vi "HP81110A Transfer String Into Memory.vi"(8 "error in (no error)":errorcluster, 9 "String":string, 10 "Channel (1:Channel 1)":T1(ring)=enum."Channel 1", 11 "VISA session":refnum<visa-resource-name>) -> (0 "error out":errorcluster, 2 "length":i32, 3 "dup VISA session":refnum<visa-resource-name>)   [LabVIEW 2023]
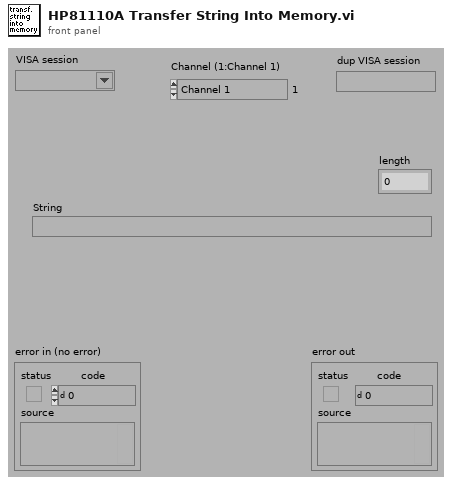
[diagram p1: front panel]
types:
  T1 = enum16{"Channel All ", "Channel 1", "Channel 2", "Channel 3", "Channels Combined"}
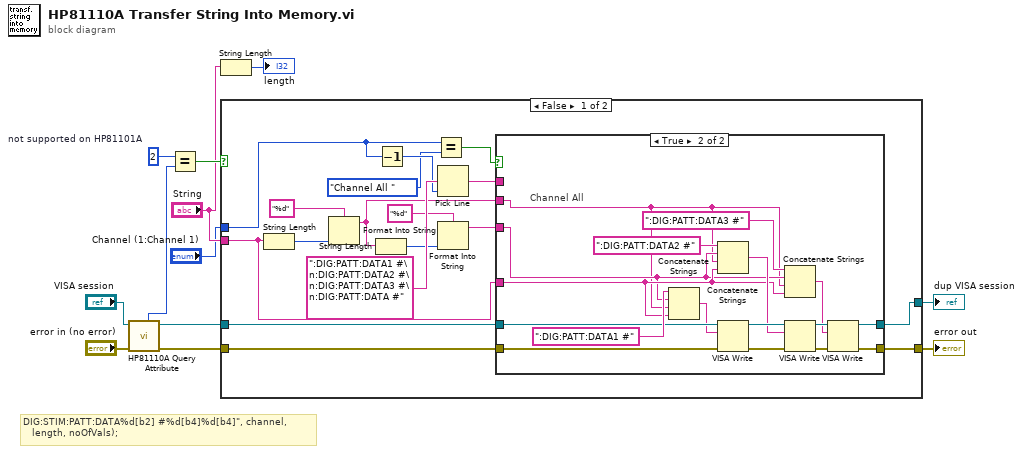
[diagram p0: block diagram]
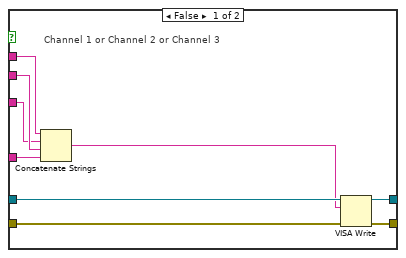
[diagram p2: hidden frame]
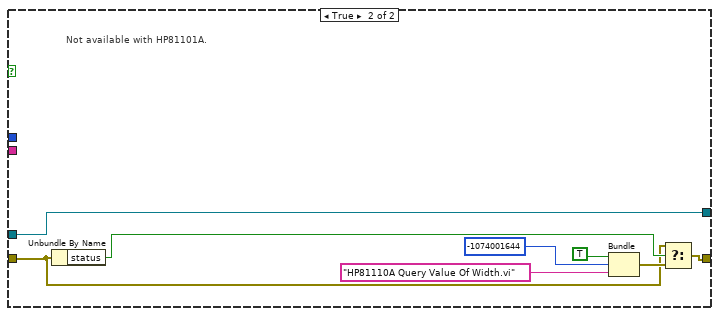
[diagram p3: hidden frame]
diagram:
  w11 = u32 2  # not supported on HP81101A
  # "DIG:STIM:PATT:DATA%d[b2] #%d[b4]%d[b4]\", channel,\n\t\t\tlength, noOfVals);"
  n1 = call "HP81110A Query Attribute.vi"("error in (no error)"="error in (no error)", "VISA session"="VISA session") -> ("error out"=w9:errorcluster, "dup VISA session"=w10:refnum<visa-resource-name>, "Instr Version"=w12:u32)  [unwired: 7 out]
  n2 = Equal?(x=w11, y=w12) -> (x = y?=w8:bool)
  n3 = String Length(string="String") -> (length=→"length":i32)
  n4 = case shown="False" w8 {
    tunnel: w10 -> [w19 w58]
    tunnel: [w16 w58] -> w7
    tunnel: w9 -> [w18 w56]
    tunnel: "Channel (1:Channel 1)" -> [w21 _]
    tunnel: [w17 w57] -> w6
    tunnel: "String" -> [w15 _]
    frame False {
      n5 = String Length(string=w15) -> (length=w14:i32)
      n6 = Format Into String(format string="%d", w14) -> (resulting string=w22:string)  [unwired: 2 in, 1 out]
      n7 = String Length(string=w22) -> (length=w25:i32)
      n8 = Decrement(x=w21) -> (x-1=w28:T1)
      n9 = Equal?(x=w21, y=T1."Channel All " ("x")) -> (x = y?=w20:bool)
      n10 = Pick Line(multi-line string=":DIG:PATT:DATA1 #\n:DIG:PATT:DATA2 #\n:DIG:PATT:DATA3 #\n:DIG:PATT:DATA #", line index=w28) -> (output string=w24:string)  [unwired: 1 out]
      n11 = Format Into String(format string="%d", w25) -> (resulting string=w23:string)  [unwired: 2 in, 1 out]
      n12 = case shown="True" w20 {
        tunnel: w15 -> [w38 w41]
        tunnel: w22 -> [w37 w39]
        tunnel: w23 -> [w36 w40]
        tunnel: w24 -> [w35 _]
        tunnel: w19 -> [w34 w54]
        tunnel: w18 -> [w33 w50]
        tunnel: [w32 w51] -> w16
        tunnel: [w31 w47] -> w17
        frame False {
          # "Channel 1 or Channel 2 or Channel 3"
          n13 = Concatenate Strings(w35, w36, w37, w38) -> (w30:string)
          n14 = VISA Write(VISA resource name=w34, write buffer=w30, error in (no error)=w33) -> (VISA resource name out=w32:refnum<visa-resource-name>, error out=w31:errorcluster)  [unwired: 1 out]
        }
        frame True {
          # "Channel All"
          n15 = Concatenate Strings(":DIG:PATT:DATA1 #", w40, w39, w41) -> (w46:string)
          n16 = Concatenate Strings(":DIG:PATT:DATA2 #", w40, w39, w41) -> (w44:string)
          n17 = VISA Write(VISA resource name=w54, write buffer=w46, error in (no error)=w50) -> (VISA resource name out=w53:refnum<visa-resource-name>, error out=w49:errorcluster)  [unwired: 1 out]
          n18 = Concatenate Strings(":DIG:PATT:DATA3 #", w40, w39, w41) -> (w43:string)
          n19 = VISA Write(VISA resource name=w53, write buffer=w44, error in (no error)=w49) -> (VISA resource name out=w52:refnum<visa-resource-name>, error out=w48:errorcluster)  [unwired: 1 out]
          n20 = VISA Write(VISA resource name=w52, write buffer=w43, error in (no error)=w48) -> (VISA resource name out=w51:refnum<visa-resource-name>, error out=w47:errorcluster)  [unwired: 1 out]
        }
      }
    }
    frame True {
      # "Not available with HP81101A."
      n21 = Unbundle By Name(w56) -> ("status"=w63:bool)
      n22 = Bundle("status"=TRUE, "code"=-1074001644, "source"="HP81110A Query Value Of Width.vi") -> (w59:errorcluster)  [unwired: 1 out]
      n23 = Select(t=w56, s=w63, f=w59) -> (s? t:f=w57:errorcluster)
    }
  }
  "dup VISA session" <- w7
  "error out" <- w6
